vi "Read Flow Rate Setpoint.vi"(8 "error in (no error)":errorcluster, 11 "MKS MF1 in":refnum<class "PL MKS MF1 USB.lvclass">) -> (0 "error out":errorcluster, 2 "flow rate setpoint, calibrated flow unit":dbl, 3 "MKS MF1 out":refnum<class "PL MKS MF1 USB.lvclass">)   [LabVIEW 2015, in "PL MKS MF1 USB.lvclass"]
doc: "Reads flow rate setpoint."
uses:
  PL MKS MF1 USB.lvclass
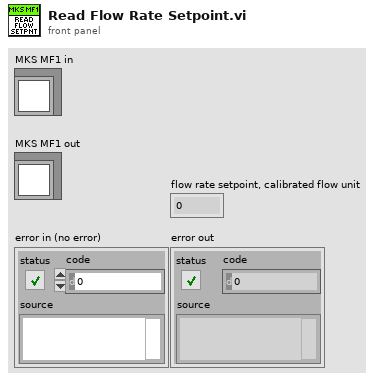
[diagram p1: front panel]
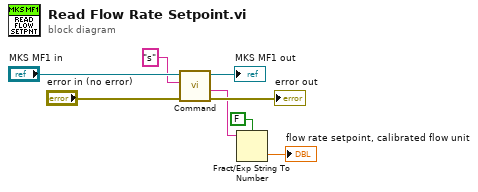
[diagram p0: block diagram]
diagram:
  n1 = call "Command.vi"("error in (no error)"="error in (no error)", "command"="s", "MKS MF1 in"="MKS MF1 in") -> ("error out"=→"error out":errorcluster, "response value"=w3:string, "MKS MF1 out"=→"MKS MF1 out":refnum<class "PL MKS MF1 USB.lvclass">)  [unwired: 5 in, 1 out]
  n2 = Fract/Exp String To Number(use system decimal point (T)=FALSE, string=w3) -> (number=→"flow rate setpoint, calibrated flow unit":dbl)  [unwired: 2 in, 1 out]
